vi "WriteRaw.vi"(0 "Array":fxp<+/-,24,4>[](array[numeric])=[0.0, 0.0, 0.0, 0.0, 0.0, 0.0, 0.0, 0.0, 0.0]) -> ()   [LabVIEW 2023]
uses:
  <vilib>/rvi/DataTransferAndStorage/Container/Common/niFpgaContainerExecOnDevCompGetState.vi
  <vilib>/rvi/Emulation/niFpgaEmulationIsFPGAContextNoSignature.vi
  <vilib>/rvi/Emulation/niFpgaSctlEmulationGetInTimedLoop.vi
  <vilib>/rvi/errors/niFpgaSetErrorForExecOnDevCompSimple.vi
  <vilib>/rvi/eio/common/nirviEmuReportErrorAndStop.vi
  <vilib>/rvi/DataTransferAndStorage/Container/Common/niFpgaContainerGetUniqueNameForEmu.vi
  <vilib>/rvi/FIFO/Fifo_Resource/nirvififoEmulationSetSize.vi
  <vilib>/rvi/FIFO/Fifo_Resource/nirviFifoEmulationQueueMgr.vi
  <instcachedir>/0/nirviFifoEmulationQueueMgr_E5CAEC123FF24DC58D834DCA3CDAA9B5.lvgen/nirviFifoEmulationQueueMgr_E5CAEC123FF24DC58D834DCA3CDAA9B5_021.vi
  <vilib>/rvi/FIFO/Fifo_Resource/nirvififoEmulationDetermineInputValidOut.vi
  <vilib>/rvi/FIFO/Fifo_Resource/nirvififoEmulationCreateLock.vi
  <vilib>/rvi/Emulation/niFpgaProcessEmulError.vi
  <vilib>/rvi/FIFO/Fifo_Resource/nirvififoEmulationObtainLock.vi
  <vilib>/rvi/FIFO/Fifo_Resource/nirvififoEmulationReleaseLock.vi
  <vilib>/rvi/occurrence/nirviWaitOnOccurrenceBase.vi
  <vilib>/rvi/errors/nirviReportUnexpectedCaseInternalError.vi
  <vilib>/rvi/errors/nirviReportUnexpectedCaseInternalError (U32).vi
  <vilib>/Utility/error.llb/Clear Errors.vi
  <vilib>/eio/utilities/niEioResolveVilibRelativePath.vi
  <vilib>/rvi/interface/RandomDataEmulation/niFpgaRandomDataHandleErrors.vi
  <vilib>/rvi/DataTransferAndStorage/Container/XNode/niFpgaContainer.xnode
  <vilib>/rvi/FIFO/Fifo_Resource/niFpgaFifoEmulationRefIn.vi
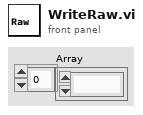
[diagram p1: front panel]
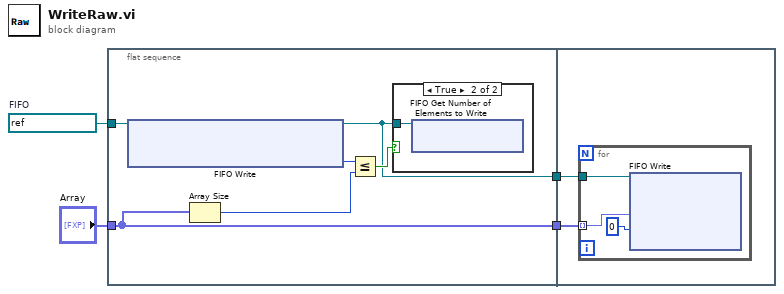
[diagram p0: block diagram]
diagram:
  w2 = refnum<k21> "RawOutput"  # FIFO
  n1 = flat-sequence {
    tunnel: "Array" -> [w10]
    tunnel: [w10] -> w3
    tunnel: w2 -> [w9]
    tunnel: [w5] -> w1
    tunnel: w3 -> [w13]
    tunnel: w1 -> [w12]
    frame #0 {
      n2 = xnode "FIFO Write"("FIFO In"=w9) -> ("Number of Elements to Write"=w8:u32, "FIFO Out"=w5:refnum<k21>)
      n3 = Array Size(array=w10) -> (size(s)=w7:i32)
      n4 = Less Or Equal?(x=w8, y=w7) -> (x <= y?=w6:bool)
      n5 = case shown="True" w6 {
        tunnel: w5 -> [_ w11]
        frame False {
        }
        frame True {
          n6 = xnode "FIFO Get Number of Elements to Write"("FIFO In"=w11) -> ()  [unwired: 1 out]
        }
      }
    }
    frame #1 {
      n7 = for {
        tunnel: w13 -> [w16] mode=indexing
        tunnel: w12 -> [w14]
        n8 = xnode "FIFO Write"("Element"=w16, "Timeout"=0, "FIFO In"=w14) -> ()  [unwired: 2 out]
      }
    }
  }
